vi "Shooter Speed Error.vi"() -> ()   [LabVIEW 2012]
panel:
  in  "Shooter Speed Error":dbl
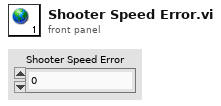
[diagram p1: front panel]
diagram:
